vi "M227_Init_v0.vi"() -> (1 "Status":bool, 2 "Position":dbl[](array[numeric]), 3 "VISA Refnum out":refnum<visa-resource-name>)   [LabVIEW 2014]
uses:
  <vilib>/Instr/_visa.llb/VISA Configure Serial Port (Instr).vi
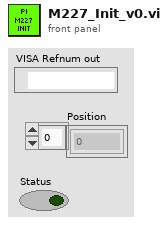
[diagram p1: front panel]
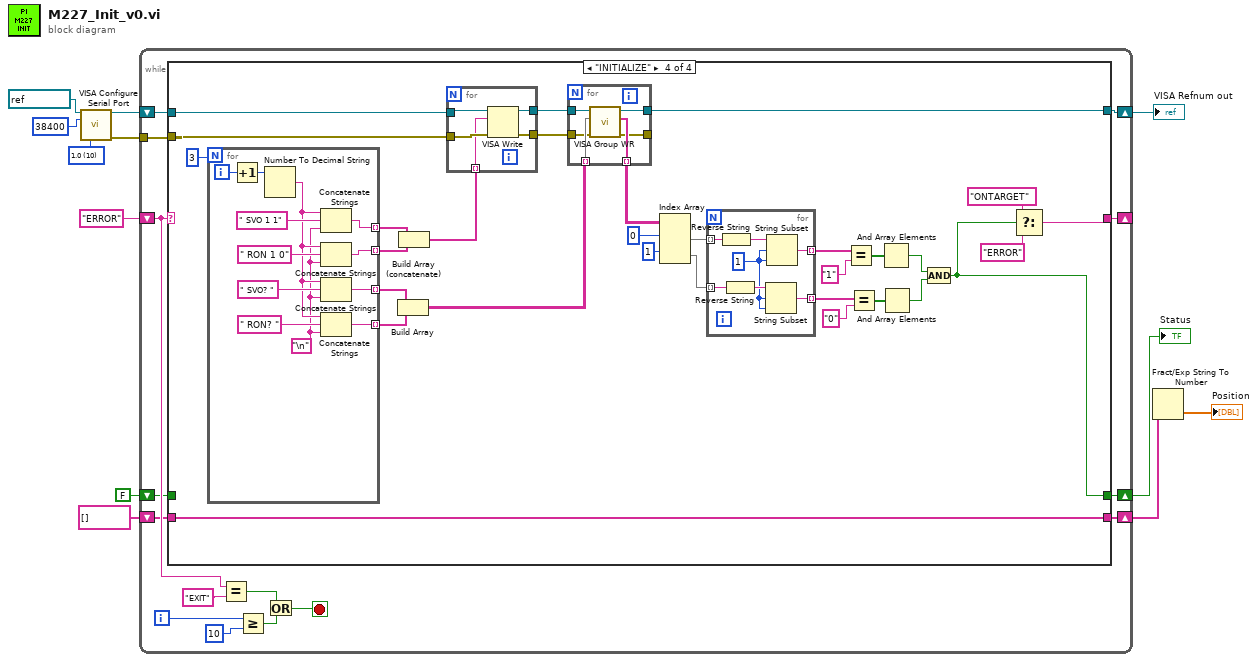
[diagram p0: block diagram]
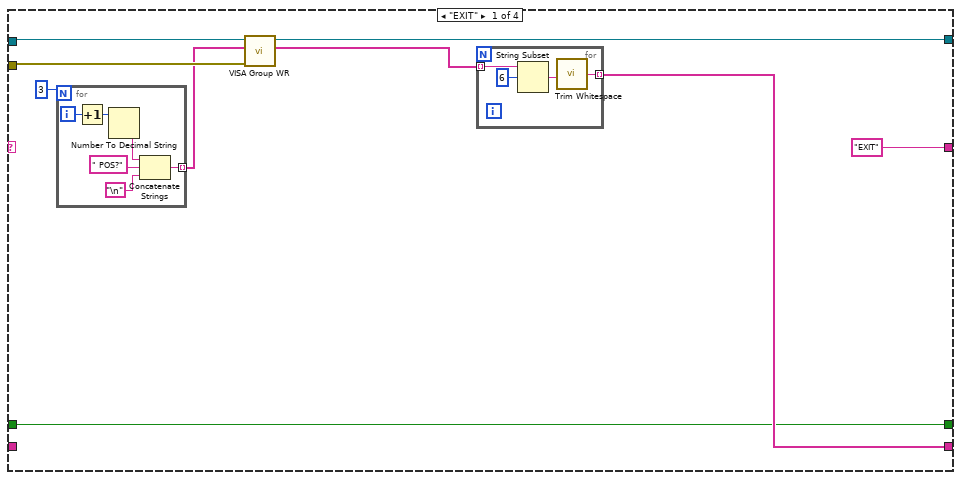
[diagram p2: hidden frame]
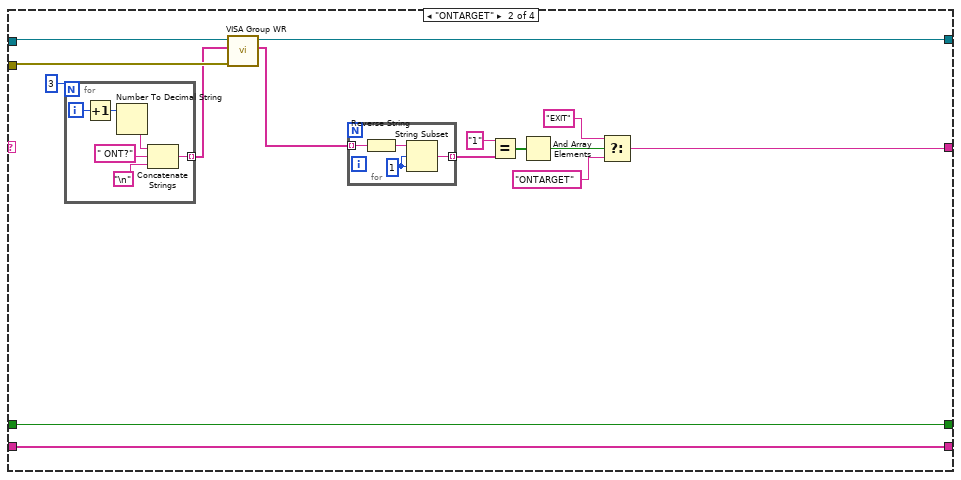
[diagram p3: hidden frame]
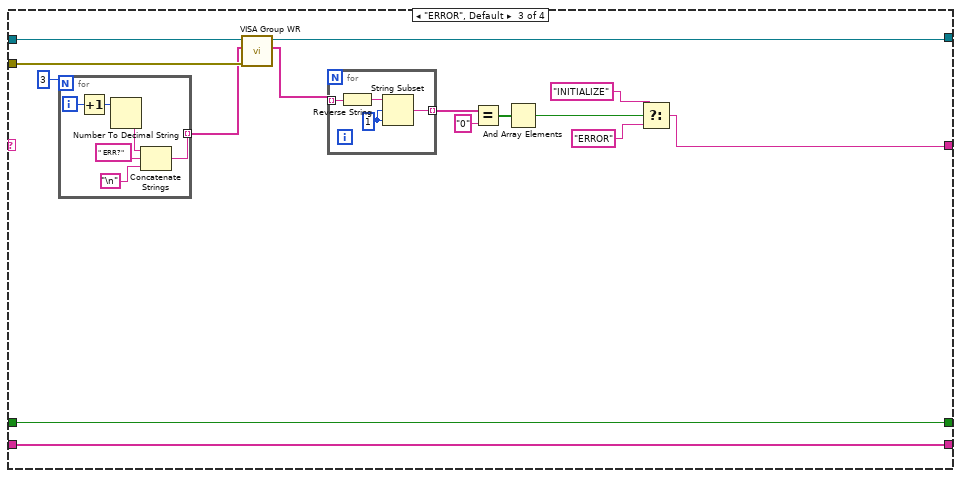
[diagram p4: hidden frame]
diagram:
  w8 = u16 10 items=["1.0"=10, "1.5"=15, "2.0"=20] ("stop bits (10: 1 bit)")
  n1 = call-poly "VISA Configure Serial Port"("VISA resource name"=refnum<visa-resource-name> "COM6", "baud rate (9600)"=u32 38400, "stop bits (10: 1 bit)"=w8) -> ("VISA resource name out"=w12:refnum<visa-resource-name>, "error out"=w9:errorcluster)  [unwired: 11 in]
  n2 = while {
    tunnel: w9 -> [w26]
    shift-right: [w25] -> _
    shift-left: "ERROR" -> [w23]
    shift-right: [w15] -> w5
    shift-left: w12 -> [w27]
    shift-right: [w16] -> w2
    shift-left: string[] [] -> [w14]
    shift-right: [w19] -> w11
    shift-left: FALSE -> [w13]
    i -> [w17]
    stop <- w21 stop-if-true
    n3 = case shown="\"INITIALIZE\"" w23 {
      tunnel: w27 -> [w35 w61 w86 w123]
      tunnel: w26 -> [w34 w60 w85 w122]
      tunnel: [w30 w50 w80 w99] -> w19
      tunnel: ["EXIT" w51 w81 w100] -> w25
      tunnel: [w32 w49 w79 w106] -> w16
      tunnel: [w31 w59 w84 w107] -> w15
      tunnel: w14 -> [_ w49 w79 w106]
      tunnel: w13 -> [w30 w50 w80 _]
      frame "EXIT" {
        n4 = for {
          N: 3 -> [_]
          tunnel: [w39] -> w29 mode=indexing
          i -> [w42]
          n5 = Increment(x=w42) -> (x+1=w41:i32)
          n6 = Number To Decimal String(number=w41) -> (decimal integer string=w40:string)  [unwired: 1 in]
          n7 = Concatenate Strings(w40, " POS?" ("string"), "\n") -> (w39:string)
        }
        n8 = call "VISA Group WR.vi"("error in (no error)"=w34, "Array in"=w29, "VISA Refnum in"=w35) -> ("Array out"=w33:string[], "VISA Refnum out"=w31:refnum<visa-resource-name>)  [unwired: 6 in, 1 out]
        n9 = for {
          tunnel: w33 -> [w46] mode=indexing
          tunnel: [w43] -> w32 mode=indexing
          n10 = String Subset(string=w46, offset (0)=6) -> (substring=w44:string)  [unwired: 1 in]
          n11 = call <vilib>:"Trim Whitespace.vi"("string"=w44) -> ("trimmed string"=w43:string)  [unwired: 1 in]
        }
      }
      frame "ONTARGET" {
        n12 = for {
          N: 3 -> [_]
          tunnel: [w63] -> w47 mode=indexing
          i -> [w67]
          n13 = Increment(x=w67) -> (x+1=w66:i32)
          n14 = Number To Decimal String(number=w66) -> (decimal integer string=w62:string)  [unwired: 1 in]
          n15 = Concatenate Strings(w62, " ONT?" ("string"), "\n") -> (w63:string)
        }
        n16 = call "VISA Group WR.vi"("error in (no error)"=w60, "Array in"=w47, "VISA Refnum in"=w61) -> ("Array out"=w56:string[], "VISA Refnum out"=w59:refnum<visa-resource-name>)  [unwired: 6 in, 1 out]
        n17 = for {
          tunnel: [w68] -> _ mode=indexing
          tunnel: [w69] -> w57 mode=indexing
          tunnel: w56 -> [w68] mode=indexing
          w70 = 1 ("length (rest)")
          n18 = Reverse String(1:w68) -> (0:w71:string)
          n19 = String Subset(string=w71, offset (0)=w70, length (rest)=w70) -> (substring=w69:string)
        }
        n20 = Equal?(x="1", y=w57) -> (x = y?=w58:bool[])
        n21 = And Array Elements(Boolean array=w58) -> (logical AND=w54:bool)
        n22 = Select(t="EXIT", s=w54, f="ONTARGET") -> (s? t:f=w51:string)
      }
      frame "ERROR", Default {
        n23 = for {
          N: 3 -> [_]
          tunnel: [w96] -> w72 mode=indexing
          i -> [w95]
          n24 = Increment(x=w95) -> (x+1=w94:i32)
          n25 = Number To Decimal String(number=w94) -> (decimal integer string=w93:string)  [unwired: 1 in]
          n26 = Concatenate Strings(w93, " ERR?" ("string"), "\n") -> (w96:string)
        }
        n27 = call "VISA Group WR.vi"("error in (no error)"=w85, "Array in"=w72, "VISA Refnum in"=w86) -> ("Array out"=w77:string[], "VISA Refnum out"=w84:refnum<visa-resource-name>)  [unwired: 6 in, 1 out]
        n28 = for {
          tunnel: [w88] -> w76 mode=indexing
          tunnel: w77 -> [w87] mode=indexing
          w90 = 1 ("length (rest)")
          n29 = Reverse String(1:w87) -> (0:w89:string)
          n30 = String Subset(string=w89, offset (0)=w90, length (rest)=w90) -> (substring=w88:string)
        }
        n31 = Equal?(x=w76, y="0") -> (x = y?=w74:bool[])
        n32 = And Array Elements(Boolean array=w74) -> (logical AND=w73:bool)
        n33 = Select(t="INITIALIZE", s=w73, f="ERROR") -> (s? t:f=w81:string)
      }
      frame "INITIALIZE" {
        n34 = for {
          N: 3 -> [_]
          tunnel: [w156] -> w105 mode=indexing
          tunnel: [w155] -> w121 mode=indexing
          tunnel: [w154] -> w120 mode=indexing
          tunnel: [w145] -> w104 mode=indexing
          i -> [w152]
          w146 = "\n"
          n35 = Increment(x=w152) -> (x+1=w153:i32)
          n36 = Number To Decimal String(number=w153) -> (decimal integer string=w147:string)  [unwired: 1 in]
          n37 = Concatenate Strings(w147, " SVO 1 1" ("string"), w146) -> (w156:string)
          n38 = Concatenate Strings(w147, " RON 1 0" ("string"), w146) -> (w145:string)
          n39 = Concatenate Strings(w147, " SVO? " ("string"), w146) -> (w155:string)
          n40 = Concatenate Strings(w147, " RON? " ("string"), w146) -> (w154:string)
        }
        n41 = Build Array(w121, w120) -> (w119:string[][])
        n42 = Build Array (concatenate)(w105, w104) -> (w103:string[])
        n43 = for {
          tunnel: w123 -> [w144]
          tunnel: w122 -> [w143]
          tunnel: [w142] -> w124
          tunnel: [w141] -> w125
          tunnel: w103 -> [w140] mode=indexing
          n44 = VISA Write(VISA resource name=w144, write buffer=w140, error in (no error)=w143) -> (VISA resource name out=w142:refnum<visa-resource-name>, error out=w141:errorcluster)  [unwired: 1 out]
        }
        n45 = for {
          tunnel: w124 -> [w139]
          tunnel: w119 -> [w138] mode=indexing
          tunnel: [w137] -> w111 mode=indexing
          tunnel: [w136] -> w107
          tunnel: w125 -> [w135]
          tunnel: [w134] -> _
          n46 = call "VISA Group WR.vi"("error in (no error)"=w135, "Array in"=w138, "VISA Refnum in"=w139) -> ("error out"=w134:errorcluster, "Array out"=w137:string[], "VISA Refnum out"=w136:refnum<visa-resource-name>)  [unwired: 6 in]
        }
        n47 = Index Array(array=w111, index (row) #1=0 ("index (row)"), index (row) #2=1 ("index (row)")) -> (element #1=w115:string[], element #2=w116:string[])  [unwired: 2 in]
        n48 = for {
          tunnel: w115 -> [w132] mode=indexing
          tunnel: [w131] -> w118 mode=indexing
          tunnel: w116 -> [w129] mode=indexing
          tunnel: [w128] -> w102 mode=indexing
          w127 = 1 ("length (rest)")
          n49 = Reverse String(1:w132) -> (0:w133:string)
          n50 = Reverse String(1:w129) -> (0:w130:string)
          n51 = String Subset(string=w130, offset (0)=w127, length (rest)=w127) -> (substring=w128:string)
          n52 = String Subset(string=w133, offset (0)=w127, length (rest)=w127) -> (substring=w131:string)
        }
        n53 = Equal?(x=w118, y="1") -> (x = y?=w117:bool[])
        n54 = Equal?(x=w102, y="0") -> (x = y?=w114:bool[])
        n55 = And Array Elements(Boolean array=w117) -> (logical AND=w98:bool)
        n56 = And Array Elements(Boolean array=w114) -> (logical AND=w97:bool)
        n57 = Compound Arithmetic op=AND(w98, w97) -> (w99:bool)
        n58 = Select(t="ONTARGET", s=w99, f="ERROR") -> (s? t:f=w100:string)
      }
    }
    n59 = Equal?(x=w23, y="EXIT") -> (x = y?=w22:bool)
    n60 = Greater Or Equal?(x=w17, y=10 ("x")) -> (x >= y?=w20:bool)
    n61 = Or(x=w22, y=w20) -> (x .or. y?=w21:bool)
  }
  "VISA Refnum out" <- w5
  "Status" <- w11
  n62 = Fract/Exp String To Number(string=w2) -> (number=→"Position":dbl[])  [unwired: 3 in, 1 out]
